vi "Close Loader Handle.vi"(8 "error in (no error)":errorcluster, 11 "Loaders":T1[](array[typedef])) -> (0 "error out":errorcluster)   [LabVIEW 2021, in "CIFPluginManager.lvclass"]
uses:
  CIFPluginManager.lvclass
  typedef/Loaders.ctl
  Common/typedef/Loader Type.ctl
  <vilib>/gRPC/LabVIEW gRPC Library/Shared/grpcId.ctl
  CIFPluginManager.lvclass/CIFPluginManager.ctl
  CIFPluginLoader/gRPC/CIF_Plugin_Loader_Client_Wrapper/CIFPluginLoaderClientWrapper.lvlib
  <vilib>/gRPC/LabVIEW gRPC Library/grpc-lvsupport-release.lvlib
  Common/Manager Common.lvlib
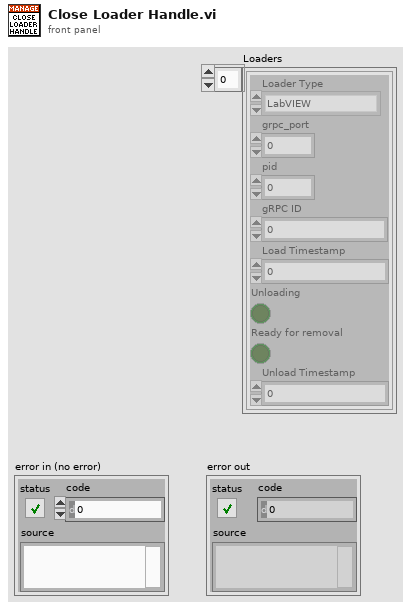
[diagram p1: front panel]
types:
  T1 = typedef "CIFPluginManager.lvclass/Loaders.ctl" = cluster{"Loader Type":T2, "grpc_port":i32, "pid":u32, "gRPC ID":T3, "Load Timestamp":i64, "Unloading":bool, "Ready for removal":bool, "Unload Timestamp":i64}
  T2 = typedef "Manager Common.lvlib/Loader Type.ctl" = enum16{"LabVIEW"}
  T3 = typedef "grpc-lvsupport-release.lvlib/grpcId.ctl" = u64
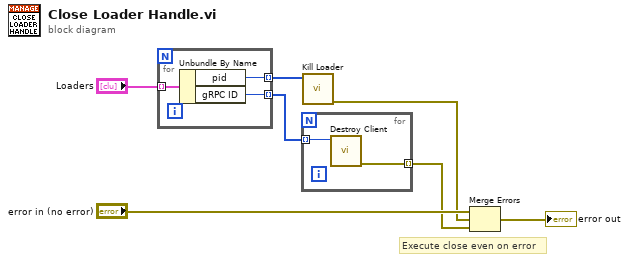
[diagram p0: block diagram]
diagram:
  # "Execute close even on error"
  n1 = for {
    tunnel: [w10] -> w4 mode=indexing
    tunnel: [w9] -> w2 mode=indexing
    tunnel: "Loaders" -> [w8] mode=indexing
    n2 = Unbundle By Name(w8) -> ("pid"=w9:u32, "gRPC ID"=w10:T3)
  }
  n3 = for {
    tunnel: [w12] -> w5 mode=indexing
    tunnel: w4 -> [w11] mode=indexing
    n4 = call "Destroy Client.vi"("gRPC ID"=w11) -> ("error out"=w12:errorcluster)  [unwired: 10 in]
  }
  n5 = call "Kill Loader.vi"("PIDs"=w2) -> ("error out"=w3:errorcluster)  [unwired: 8 in, 2 out]
  n6 = Merge Errors("error in (no error)", w3, w5) -> (→"error out":errorcluster)
